vi "TrapsMachMitteln-15-07-17.vi"(0 "FPGA VI Reference In":refnum<k20>, 1 "Traps/MachKoeff2":dbl[](array[numeric]), 2 "Traps/MachKoeff1":dbl[](array[numeric]), 3 "Traps/MachKoeff0":dbl[](array[numeric]), 4 "error in":errorcluster) -> (5 "error out":errorcluster)   [LabVIEW 2017]
uses:
  <vilib>/Utility/error.llb/Error Cluster From Error Code.vi
  <vilib>/rvi/errors/niLvFpgaAdjustHostInterfaceError.vi
  GVTrapsMachs.vi
  <vilib>/rvi/interface/nirviReadWriteControl/nirviReadWriteControl.xnode
  FPGA Bitfiles/HAGAR-V_FPGATarget_FPGA-Programm-05_gdVwCsZS6sg.lvbitx
  FPGA/FPGA-Programm-05-17.vi
  NiFpgaLv.dll
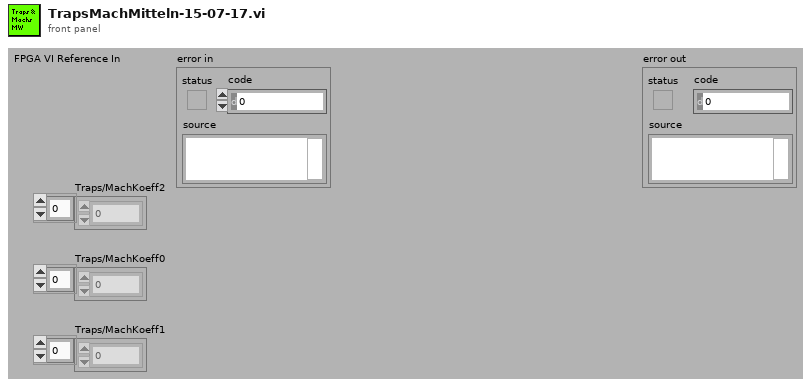
[diagram p1: front panel]
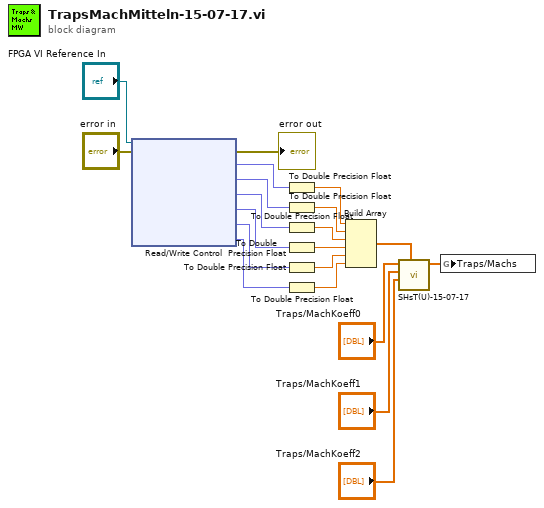
[diagram p0: block diagram]
diagram:
  n1 = xnode "Read/Write Control"("FPGA-VI-Referenz (Eingang)"="FPGA VI Reference In", "Fehler (Eingang)"="error in") -> ("Fehler (Ausgang)"=→"error out":errorcluster, "MesswertTrap1"=w20:fxp<+/-,26,5>, "MesswertTrap2"=w19:fxp<+/-,26,5>, "U[V]PreMach1"=w18:fxp<+/-,26,5>, "U[V]PreMach2"=w17:fxp<+/-,26,5>, "U[V]MainMach1"=w16:fxp<+/-,26,5>, "U[V]MainMach2"=w15:fxp<+/-,26,5>)  [unwired: 1 out]
  n2 = To Double Precision Float(number=w20) -> (double precision float=w7:dbl)
  n3 = To Double Precision Float(number=w19) -> (double precision float=w6:dbl)
  n4 = To Double Precision Float(number=w18) -> (double precision float=w14:dbl)
  n5 = To Double Precision Float(number=w17) -> (double precision float=w13:dbl)
  n6 = To Double Precision Float(number=w16) -> (double precision float=w12:dbl)
  n7 = To Double Precision Float(number=w15) -> (double precision float=w11:dbl)
  n8 = Build Array(w7, w6, w14, w13, w12, w11) -> (w5:dbl[])
  n9 = call "SHsT(U)-15-07-17.vi"("SpannungenSH[V]"=w5, "Traps/MachKoeff2"="Traps/MachKoeff2", "Traps/MachKoeff1"="Traps/MachKoeff1", "Traps/MachKoeff0"="Traps/MachKoeff0") -> ("TemperaturenSH[°C]"=w1:dbl[])  [unwired: 7 in]
  n10 = global write "GVTrapsMachs.vi" "Traps/Machs"(w1) -> ()
